vi "cmd_vel_cal.vi"(8 "P3AT_Panel":T1={"max_vel"=0.49056603773584906, "max_rot"=0.5094339622641509, "Control_Mode"=enum."Joy"} {"max_rot" scale=0.0..1.0; "max_vel" scale=0.0..1.0}, 9 "XBOX_Control":T2) -> (3 "vel_cal":cluster{"rot_z":dbl, "lin_x":dbl})   [LabVIEW 2014]
uses:
  ctl/XBOX_Control.ctl
  <vilib>/MakerHub/Xbox-One-Controller/Private/Type Defs/Indicators/All Buttons Visual.ctl
  <vilib>/MakerHub/Xbox-One-Controller/Private/Type Defs/Indicators/A.ctl
  <vilib>/MakerHub/Xbox-One-Controller/Private/Type Defs/Indicators/B.ctl
  <vilib>/MakerHub/Xbox-One-Controller/Private/Type Defs/Indicators/X.ctl
  <vilib>/MakerHub/Xbox-One-Controller/Private/Type Defs/Indicators/Y.ctl
  <vilib>/MakerHub/Xbox-One-Controller/Private/Type Defs/Indicators/Left Bumper.ctl
  <vilib>/MakerHub/Xbox-One-Controller/Private/Type Defs/Indicators/Right Bumper.ctl
  <vilib>/MakerHub/Xbox-One-Controller/Private/Type Defs/Indicators/View.ctl
  <vilib>/MakerHub/Xbox-One-Controller/Private/Type Defs/Indicators/Menu.ctl
  <vilib>/MakerHub/Xbox-One-Controller/Private/Type Defs/Indicators/Thumbstick.ctl
  <vilib>/MakerHub/Xbox-One-Controller/Private/Type Defs/Indicators/All Axis Data.ctl
  <vilib>/MakerHub/Xbox-One-Controller/Private/Type Defs/Indicators/DPad Enum.ctl
  ctl/P3AT_Panel.ctl
  <vilib>/MakerHub/Xbox-One-Controller/LMH-Xbox-One-Controller.lvlib
panel:
  out "lin_x":dbl
  out "rot_z":dbl
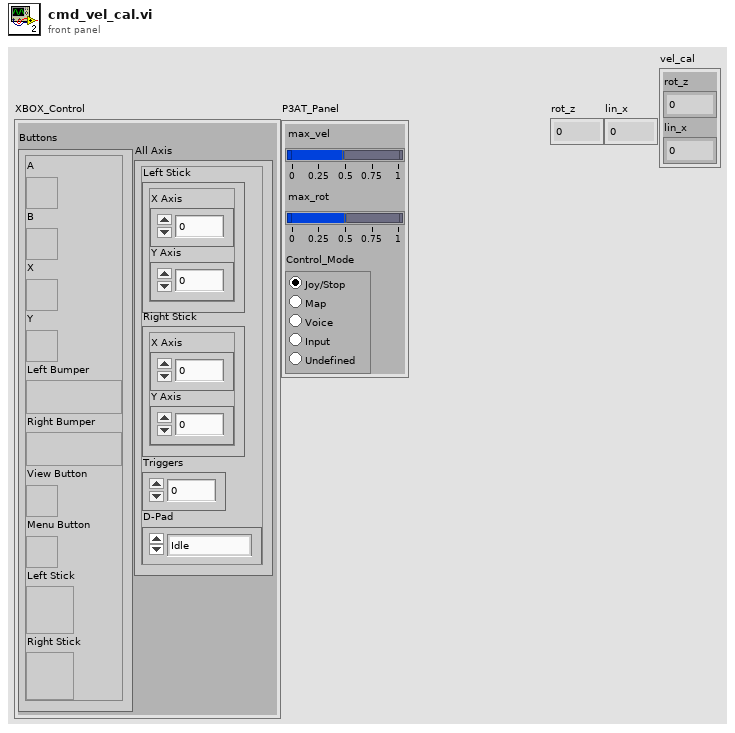
[diagram p1: front panel]
types:
  T1 = typedef "P3AT_Panel.ctl" = cluster{"max_vel":dbl, "max_rot":dbl, "Control_Mode":enum32{"Joy", "Map", "Voice", "Input", "Undefined"}}
  T2 = typedef "XBOX_Control.ctl" = cluster{"Buttons":T3, "All Axis":T13}
  T3 = typedef "LMH-Xbox-One-Controller.lvlib/All Buttons Visual.ctl" = cluster{"A":T4, "B":T5, "X":T6, "Y":T7, "Left Bumper":T8, "Right Bumper":T9, "View Button":T10, "Menu Button":T11, "Left Stick":T12, "Right Stick":T12}
  T4 = typedef "LMH-Xbox-One-Controller.lvlib/A.ctl" = bool
  T5 = typedef "LMH-Xbox-One-Controller.lvlib/B.ctl" = bool
  T6 = typedef "LMH-Xbox-One-Controller.lvlib/X.ctl" = bool
  T7 = typedef "LMH-Xbox-One-Controller.lvlib/Y.ctl" = bool
  T8 = typedef "LMH-Xbox-One-Controller.lvlib/Left Bumper.ctl" = bool
  T9 = typedef "LMH-Xbox-One-Controller.lvlib/Right Bumper.ctl" = bool
  T10 = typedef "LMH-Xbox-One-Controller.lvlib/View.ctl" = bool
  T11 = typedef "LMH-Xbox-One-Controller.lvlib/Menu.ctl" = bool
  T12 = typedef "LMH-Xbox-One-Controller.lvlib/Thumbstick.ctl" = bool
  T13 = typedef "LMH-Xbox-One-Controller.lvlib/All Axis Data.ctl" = cluster{"Left Stick":cluster{"X Axis":i32, "Y Axis":i32}, "Right Stick":cluster{"X Axis":i32, "Y Axis":i32}, "Triggers":i32, "D-Pad":T14}
  T14 = typedef "LMH-Xbox-One-Controller.lvlib/DPad Enum.ctl" = enum16{"Idle", "Up", "Up / Right", "Right", "Down / Right", "Down", "Down / Left", "Left", "Up / Left"}
  T15 = enum32{"Joy", "Map", "Voice", "Input", "Undefined"}
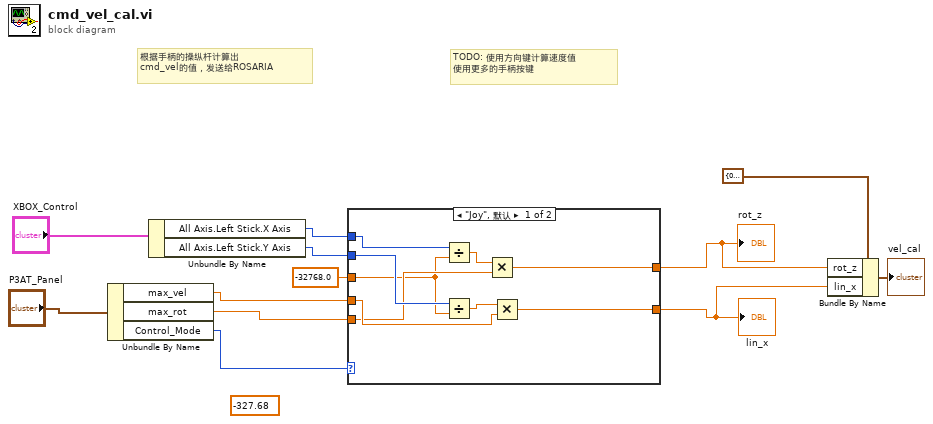
[diagram p0: block diagram]
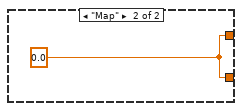
[diagram p2: hidden frame]
diagram:
  (unwired) -327.68
  # "TODO: 使用方向键计算速度值\n使用更多的手柄按键"
  # "根据手柄的操纵杆计算出\ncmd_vel的值，发送给ROSARIA"
  n1 = Unbundle By Name("P3AT_Panel") -> ("max_vel"=w10:dbl, "max_rot"=w9:dbl, "Control_Mode"=w7:T15)
  n2 = Unbundle By Name("XBOX_Control") -> ("All Axis.Left Stick.X Axis"=w12:i32, "All Axis.Left Stick.Y Axis"=w11:i32)
  n3 = case shown="\"Joy\", 默认" w7 {
    tunnel: w12 -> [w20 _]
    tunnel: w11 -> [w19 _]
    tunnel: w10 -> [w17 _]
    tunnel: w9 -> [w16 _]
    tunnel: -32768.0 -> [w15 _]
    tunnel: [w14 w22] -> w4
    tunnel: [w13 w22] -> w3
    frame "Joy", Default {
      n4 = Divide(x=w20, y=w15) -> (x/y=w21:dbl)
      n5 = Divide(x=w19, y=w15) -> (x/y=w18:dbl)
      n6 = Multiply(x=w21, y=w16) -> (x*y=w14:dbl)
      n7 = Multiply(x=w18, y=w17) -> (x*y=w13:dbl)
    }
    frame "Map" {
      w22 = 0.0
    }
  }
  "rot_z" <- w4
  "lin_x" <- w3
  n8 = Bundle By Name(cluster=cluster{"rot_z":dbl, "lin_x":dbl} {"rot_z"=0.0, "lin_x"=0.0} ("vel_cal"), "rot_z"=w4, "lin_x"=w3) -> (→"vel_cal":cluster{"rot_z":dbl, "lin_x":dbl})
